vi "cwlaserControl.vi"() -> ()   [LabVIEW 2017]
panel:
  in  "STOP":bool
  in  "cwlaser1 on/off":bool
  in  "cwlaser1 power":dbl
  in  "cwlaser1 RS232 Serial Port":refnum<visa-resource-name>="COM1"
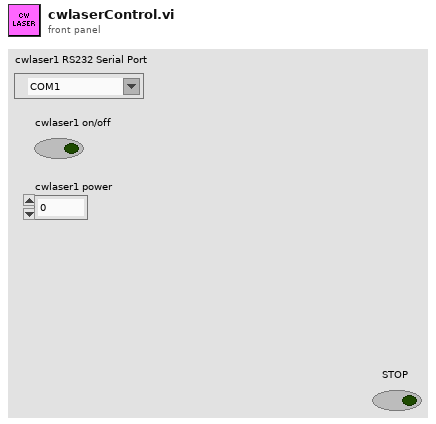
[diagram p1: front panel]
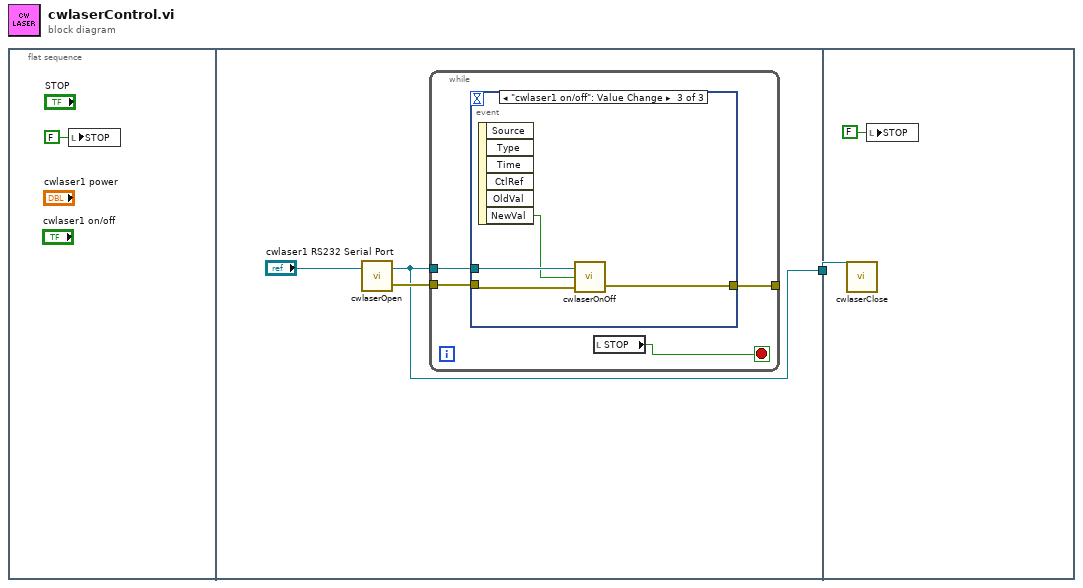
[diagram p0: block diagram]
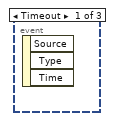
[diagram p2: hidden frame]
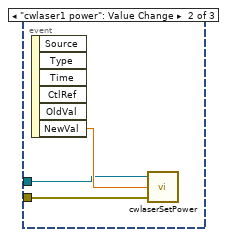
[diagram p3: hidden frame]
diagram:
  n1 = flat-sequence {
    tunnel: [w3] -> w1
    tunnel: w1 -> [w18]
    frame #0 {
      n2 = local write "STOP"(FALSE ("STOP")) -> ()
    }
    frame #1 {
      n3 = call "cwlaserOpen.vi"("cwlaser RS232 Serial Port"="cwlaser1 RS232 Serial Port") -> ("error out"=w4:errorcluster, "cwlaser"=w3:refnum<visa-resource-name>)  [unwired: 1 in]
      n4 = while {
        tunnel: w3 -> [w9]
        tunnel: w4 -> [w8]
        tunnel: [w6] -> _
        stop <- w7 stop-if-true
        n5 = event shown="[2] \"cwlaser1 on/off\": Value Change" {
          selector: _ -> [_ _ _]
          dyn-events: _ -> [_ _ _]
          timeout: _ -> [_ _ _]
          tunnel: w9 -> [_ w11 w16]
          tunnel: w8 -> [_ w10 w15]
          tunnel: [_ _ w13] -> w6
          event Timeout {
            n6 = event-data() -> ()  [unwired: 1 in, 3 out]
          }
          event "cwlaser1 power": Value Change {
            n7 = event-data() -> ("NewVal"=w12:dbl)  [unwired: 1 in, 5 out]
            n8 = call "cwlaserSetPower.vi"("error in"=w10, "power (mW)"=w12, "cwlaser in"=w11) -> ()  [unwired: 3 out]
          }
          event "cwlaser1 on/off": Value Change {
            n9 = event-data() -> ("NewVal"=w14:bool)  [unwired: 1 in, 5 out]
            n10 = call "cwlaserOnOff.vi"("error in"=w15, "Laser On/Off"=w14, "cwlaser in"=w16) -> ("error out"=w13:errorcluster)  [unwired: 1 out]
          }
        }
        n11 = local read "STOP"() -> (w7:bool)
      }
    }
    frame #2 {
      n12 = call "cwlaserClose.vi"("cwlaser in"=w18) -> ()  [unwired: 1 in, 1 out]
      n13 = local write "STOP"(FALSE ("STOP")) -> ()
    }
  }
